vi "Modelos.vi"() -> ()   [LabVIEW 2017]
uses:
  <vilib>/picture/3D Picture Control/NI_3D Picture Control.lvlib
panel:
  in  "Rotate":cluster{"X":dbl, "Y":dbl, "Z":dbl, "Angulo":dbl}
  in  "Escala":cluster{"X":dbl, "Y":dbl, "Z":dbl}
  in  "Trasladar":cluster{"X":dbl, "Y":dbl, "Z":dbl}
  out "text":string[](array[string])
  out "3D Picture":refnum<vi>(3d-picture)
  in  "File Path Control":path
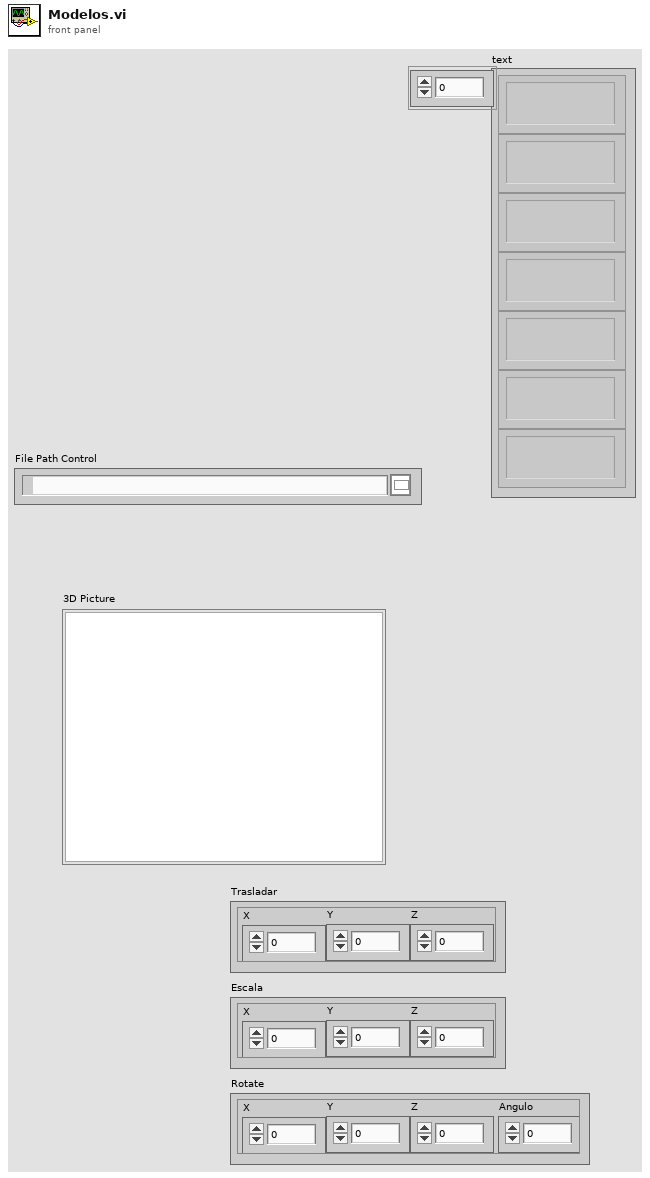
[diagram p1: front panel]
types:
  T1 = enum16{"open", "replace", "create", "open or create", "replace or create", "replace or create with confirmation"}
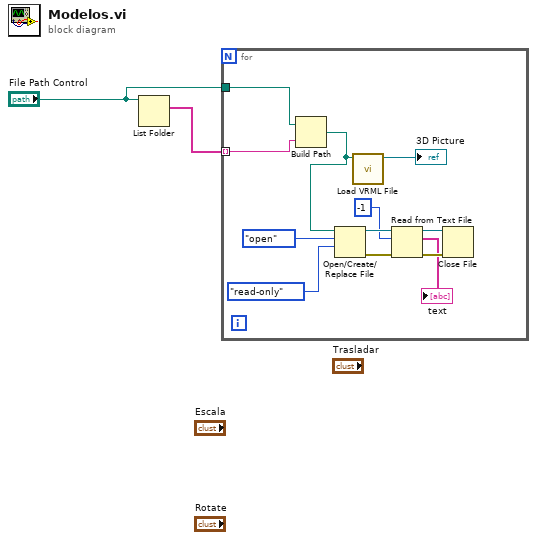
[diagram p0: block diagram]
diagram:
  n1 = List Folder(path="File Path Control") -> (filenames=w2:string[])  [unwired: 3 in, 3 out]
  n2 = for {
    tunnel: w2 -> [w13] mode=indexing
    tunnel: "File Path Control" -> [w14]
    n3 = Build Path(base path=w14, name or relative path=w13) -> (appended path=w5:path)
    n4 = Open/Create/Replace File(file path (use dialog)=w5, operation (0:open)=T1."open", access (0:read/write)=enum16{"read/write", "read-only", "write-only"}."read-only") -> (refnum out=w8:refnum<file>, error out=w11:errorcluster)  [unwired: 3 in, 1 out]
    n5 = call <vilib>:"Load VRML File.vi"("Path"=w5) -> ("Scene:Read Scene File"=→"3D Picture":refnum<vi>)  [unwired: 9 in, 1 out]
    n6 = Read from Text File(file (use dialog)=w8, count=-1, error in=w11) -> (refnum out=w9:refnum<file>, text=→"text":string[], error out=w10:errorcluster)  [unwired: 1 in, 1 out]
    n7 = Close File(refnum=w9, error in=w10) -> ()  [unwired: 2 out]
  }
